vi "circular_fitting_particle(subVI).vi"(8 "error in (no error)":errorcluster, 10 "Image Dst":T1, 11 "Image Src":T1) -> (0 "error out":errorcluster, 2 "Array":T2(array[cluster]), 3 "Image Out":T1)   [LabVIEW 2020]
doc: "Trova i cerchi pieni all'interno dell'immagine e disegna il contorno. Fornisce in uscita l'array dei cerchi.\n\nIMAGE SOURCE: immagine binarizzata.\nIMAGE DESTINATION: dove va a disegnare l'immagine."
uses:
  <vilib>/vision/Image Controls.llb/IMAQ Image.ctl
  <vilib>/vision/NI_Vision_Development_Module.lvlib
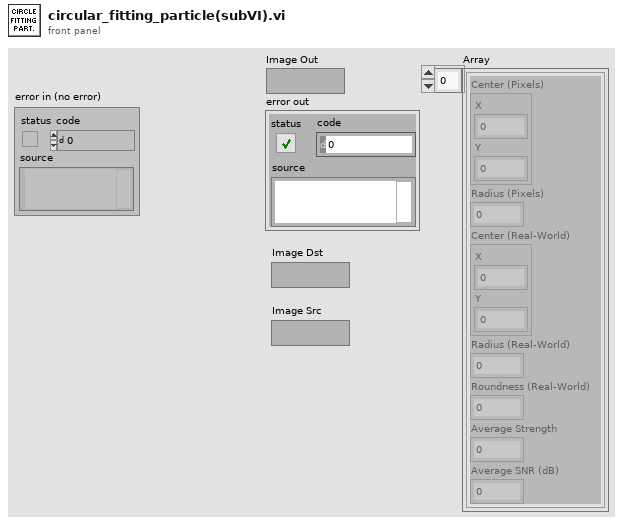
[diagram p1: front panel]
types:
  T1 = typedef "IMAQ Image.ctl" = refnum<image>
  T2 = cluster{"Center (Pixels)":cluster{"X":sgl, "Y":sgl}, "Radius (Pixels)":dbl, "Center (Real-World)":cluster{"X":sgl, "Y":sgl}, "Radius (Real-World)":dbl, "Roundness (Real-World)":dbl, "Average Strength":dbl, "Average SNR (dB)":dbl}[]
  T3 = typedef "IMAQ Circle" = cluster{"Center X":i32, "Center Y":i32, "Inner Radius":i32, "Outer Radius":i32, "Start Angle":dbl, "End Angle":dbl}
  T4 = cluster{"Area":dbl, "Number of Holes":dbl, "Bounding Rect":cluster{"Left":dbl, "Top":dbl, "Right":dbl, "Bottom":dbl}, "Center of Mass":cluster{"X":dbl, "Y":dbl}, "Orientation":dbl, "Dimensions":cluster{"Width":dbl, "Height":dbl}}[]
  T5 = typedef "ROI Descriptor" = cluster{"Global Rectangle":i32[], "Contours":cluster{"ID":enum32{"External", "Internal"}, "Type":u32, "Coordinates":i32[]}[]}
  T6 = cluster{"Center (Pixels)":cluster{"X":sgl, "Y":sgl}, "Radius (Pixels)":dbl, "Center (Real-World)":cluster{"X":sgl, "Y":sgl}, "Radius (Real-World)":dbl, "Roundness (Real-World)":dbl, "Average Strength":dbl, "Average SNR (dB)":dbl}
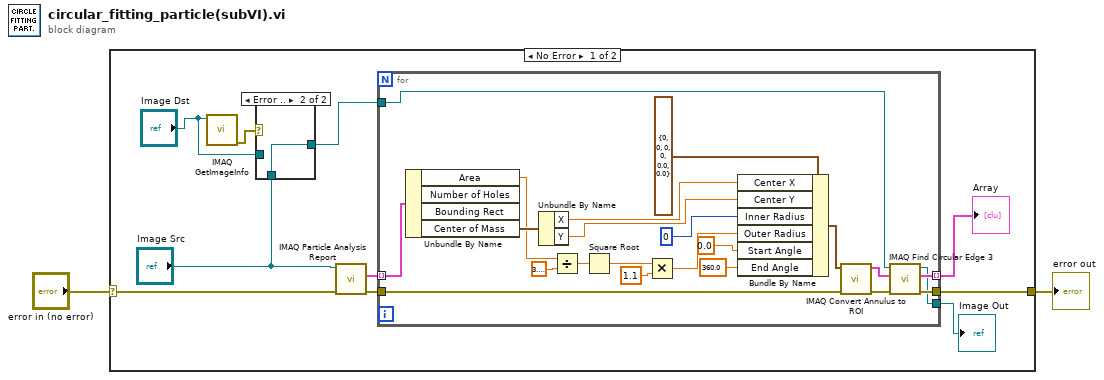
[diagram p0: block diagram]
diagram:
  n1 = case shown="No Error" "error in (no error)" {
    selector: "error in (no error)" -> [w7 w37]
    tunnel: [w9 w37] -> w2
    frame No Error {
      n2 = call "IMAQ GetImageInfo"("Image"="Image Dst") -> ("error out"=w6:errorcluster)  [unwired: 3 in, 7 out]
      n3 = case shown="Error .." w6 {
        tunnel: [w13 w14] -> w4
        tunnel: "Image Src" -> [_ w14]
        tunnel: "Image Dst" -> [w13 _]
        frame No Error {
        }
        frame Error {
        }
      }
      n4 = call "IMAQ Particle Analysis Report"("error in (no error)"=w7, "Image"="Image Src") -> ("error out"=w11:errorcluster, "Particle Reports (Pixels)"=w12:T4)  [unwired: 4 in, 4 out]
      n5 = for {
        tunnel: w12 -> [w36] mode=indexing
        tunnel: w11 -> [w33]
        tunnel: [w32] -> w9
        tunnel: [w31] -> w8 mode=indexing
        tunnel: [w30] -> w10
        tunnel: w4 -> [w29]
        n6 = Unbundle By Name(w36) -> ("Area"=w22:dbl, "Center of Mass"=w28:cluster{"X":dbl, "Y":dbl})  [unwired: 2 out]
        n7 = Unbundle By Name(w28) -> ("X"=w26:dbl, "Y"=w25:dbl)
        n8 = Divide(x=w22, y=3.141592653589793) -> (x/y=w20:dbl)
        n9 = Square Root(x=w20) -> (sqrt(x)=w19:dbl)
        n10 = Multiply(x=w19, y=1.1) -> (x*y=w17:dbl)
        n11 = Bundle By Name(cluster=T3 {"Center X"=0, "Center Y"=0, "Inner Radius"=0, "Outer Radius"=0, "Start Angle"=0.0, "End Angle"=0.0} ("Annulus"), "Center X"=w26, "Center Y"=w25, "Inner Radius"=0, "Outer Radius"=w17, "Start Angle"=0.0, "End Angle"=360.0) -> (w24:T3)
        n12 = call "IMAQ Convert Annulus to ROI"("error in (no error)"=w33, "Annulus"=w24) -> ("error out"=w34:errorcluster, "ROI Descriptor"=w35:T5)  [unwired: 7 in]
        n13 = call "IMAQ Find Circular Edge 3"("error in (no error)"=w34, "ROI Descriptor"=w35, "Image"=w29) -> ("error out"=w32:errorcluster, "Fitted Circle"=w31:T6, "Image Out"=w30:T1)  [unwired: 4 in, 2 out]
      }
      "Image Out" <- w10
      "Array" <- w8
    }
    frame Error {
    }
  }
  "error out" <- w2
